vi "Read Block.vi"(8 "error in (no error)":errorcluster, 11 "VisaComms in":refnum<class "VisaComms.lvclass">) -> (0 "error out":errorcluster, 2 "Block":string, 3 "VisaComms out":refnum<class "VisaComms.lvclass">, 5 "Buffer":string)   [LabVIEW 2024, in "CTI.lvlib" / "VisaComms.lvclass"]
uses:
  VisaComms.lvclass
  VisaComms.lvclass/VisaComms.ctl
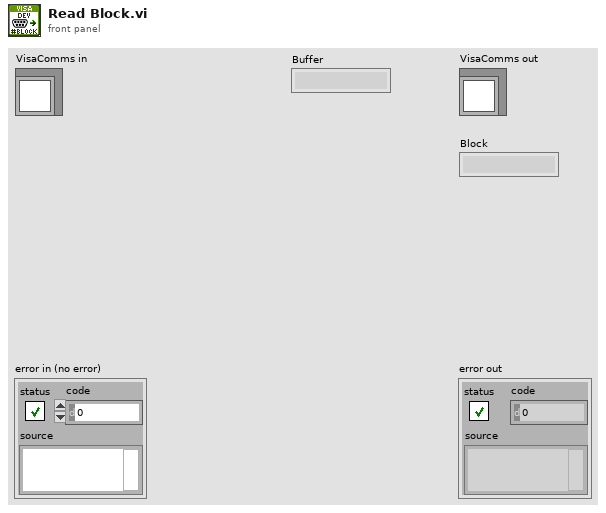
[diagram p1: front panel]
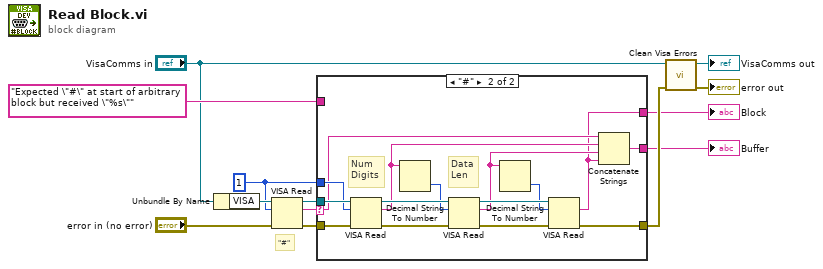
[diagram p0: block diagram]
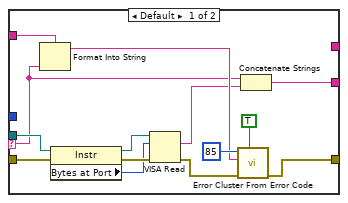
[diagram p2: hidden frame]
diagram:
  w4 = u32 1 ("byte count")
  # "\"#\""
  n1 = Unbundle By Name("VisaComms in") -> ("VISA"=w7:refnum<visa-resource-name>)
  n2 = VISA Read(VISA resource name=w7, byte count=w4, error in (no error)="error in (no error)") -> (VISA resource name out=w11:refnum<visa-resource-name>, read buffer=w12:string, error out=w10:errorcluster)  [unwired: 1 out]
  n3 = case shown="\"#\"" w12 {
    selector: w12 -> [w15 w32]
    tunnel: w11 -> [w21 w42]
    tunnel: w10 -> [w20 w41]
    tunnel: w4 -> [_ w40]
    tunnel: [w23 w33] -> w13
    tunnel: [_ w29] -> w5
    tunnel: "Expected \"#\" at start of arbitrary block but received \"%s\"" -> [w22 _]
    tunnel: [w14 w28] -> w3
    frame Default {
      n4 = Format Into String(format string=w22, w15) -> (resulting string=w25:string)  [unwired: 2 in, 1 out]
      n5 = property class="Instr"(reference=w21, error in=w20) -> (reference out=w19:refnum<visa-resource-name>, error out=w27:errorcluster, "Bytes at Port"=w18:u32)
      n6 = VISA Read(VISA resource name=w19, byte count=w18, error in (no error)=w27) -> (read buffer=w16:string, error out=w17:errorcluster)  [unwired: 2 out]
      n7 = call <vilib>:"Error Cluster From Error Code.vi"("show call chain? (False)"=TRUE, "error in (no error)"=w17, "error message (\"\")"=w25, "error code (0)"=85) -> ("error out"=w23:errorcluster)  [unwired: 5 in]
      n8 = Concatenate Strings(w15, w16) -> (w14:string)
    }
    frame "#" {
      # "Data\nLen"
      # "Num\nDigits"
      n9 = VISA Read(VISA resource name=w42, byte count=w40, error in (no error)=w41) -> (VISA resource name out=w39:refnum<visa-resource-name>, read buffer=w31:string, error out=w38:errorcluster)  [unwired: 1 out]
      n10 = Decimal String To Number(string=w31) -> (number=w37:i32)  [unwired: 2 in, 1 out]
      n11 = VISA Read(VISA resource name=w39, byte count=w37, error in (no error)=w38) -> (VISA resource name out=w36:refnum<visa-resource-name>, read buffer=w30:string, error out=w35:errorcluster)  [unwired: 1 out]
      n12 = Decimal String To Number(string=w30) -> (number=w34:i32)  [unwired: 2 in, 1 out]
      n13 = VISA Read(VISA resource name=w36, byte count=w34, error in (no error)=w35) -> (read buffer=w29:string, error out=w33:errorcluster)  [unwired: 2 out]
      n14 = Concatenate Strings(w32, w31, w30, w29) -> (w28:string)
    }
  }
  "Block" <- w5
  "Buffer" <- w3
  n15 = call "Clean Visa Errors.vi"("error in (no error)"=w13, "VisaComms in"="VisaComms in") -> ("error out"=→"error out":errorcluster, "VisaComms out"=→"VisaComms out":refnum<class "VisaComms.lvclass">)  [unwired: 8 in]
